vi "rs3 delete3.vi"(8 "error in (no error)":errorcluster, 11 "device":u64) -> (0 "error out":errorcluster)   [LabVIEW 2019, in "libRealSense3.lvlib"]
doc: "Delete the device after the sensor has been stopped, closed, deleted."
uses:
  libRealSense3.lvlib
  realsense2.dll
panel:
  # "RS3 Delete Device"
  # "(C) Intel Corp. 2017, AGJ"
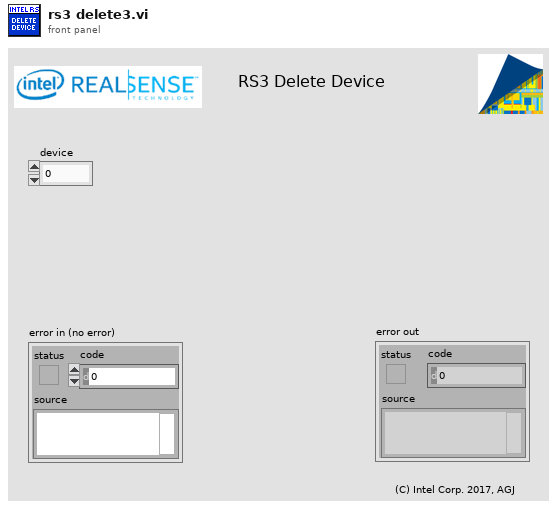
[diagram p1: front panel]
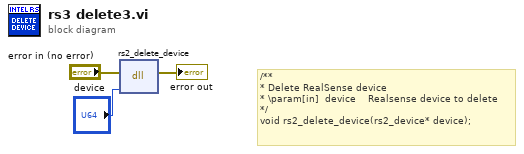
[diagram p0: block diagram]
diagram:
  # "/**\n* Delete RealSense device\n* \\param[in]  device    Realsense device to delete\n*/\nvoid rs2_delete_device(rs2_device* device);"
  n1 = dll-call lib="C:/SmartekVision/Projects/RS-D4-ETH/Software/RS-SDK/wrappers/labview/realsense2.dll" fn="rs2_delete_device"(error in="error in (no error)", "device"="device") -> (error out=→"error out":errorcluster)  [unwired: 4 in, 1 out]
